vi "write_access_codes_to_file.vi"(8 "error in":errorcluster, 10 "Codes":cluster{"Access":string, "Refresh":string}, 11 "Paths In":cluster{"Access":path, "Refresh":path}) -> (0 "error out":errorcluster)   [LabVIEW 2016]
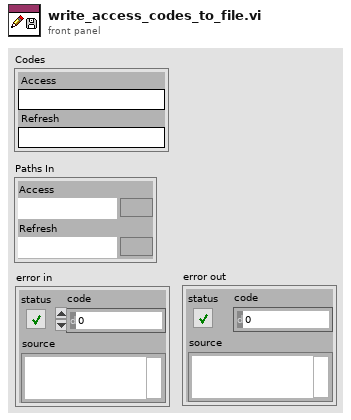
[diagram p1: front panel]
types:
  T1 = enum16{"open", "replace", "create", "open or create", "replace or create", "replace or create with confirmation"}
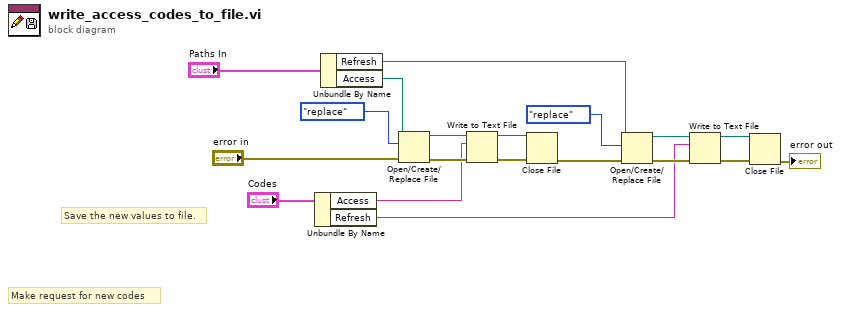
[diagram p0: block diagram]
diagram:
  # "Save the new values to file."
  # "Make request for new codes"
  n1 = Unbundle By Name("Codes") -> ("Access"=w5:string, "Refresh"=w6:string)
  n2 = Unbundle By Name("Paths In") -> ("Refresh"=w8:path, "Access"=w9:path)
  n3 = Open/Create/Replace File(file path (use dialog)=w9, error in="error in", operation (0:open)=T1."replace") -> (refnum out=w19:refnum<file>, error out=w17:errorcluster)  [unwired: 3 in, 1 out]
  n4 = Write to Text File(file (use dialog)=w19, text=w5, error in=w17) -> (refnum out=w18:refnum<file>, error out=w16:errorcluster)  [unwired: 1 in, 1 out]
  n5 = Close File(refnum=w18, error in=w16) -> (error out=w7:errorcluster)  [unwired: 1 out]
  n6 = Open/Create/Replace File(file path (use dialog)=w8, error in=w7, operation (0:open)=T1."replace") -> (refnum out=w12:refnum<file>, error out=w14:errorcluster)  [unwired: 3 in, 1 out]
  n7 = Write to Text File(file (use dialog)=w12, text=w6, error in=w14) -> (refnum out=w13:refnum<file>, error out=w15:errorcluster)  [unwired: 1 in, 1 out]
  n8 = Close File(refnum=w13, error in=w15) -> (error out=→"error out":errorcluster)  [unwired: 1 out]
